vi "I-stat example1.vi"() -> ()   [LabVIEW 2020]
uses:
  SEC Software V3.0/Labview/IVIUM/IVIUM_remdriver.lvlib
panel:
  out "Cell on":bool
  out "C off pressed":bool
  out "E OL":bool
  out "Aninput OL":bool
  out "O overload":bool
  out "Current":dbl
  out "return type":i32
  in  "uA":dbl
  out "potential":dbl
  in  "Stop":bool
  in  "Default\nCurrent range":T1(ring)=enum."100 uA"
  in  "Default Filter":T2(ring)=enum."10 kHz"
  in  "Set Stability":T3(ring)=enum."Standard"
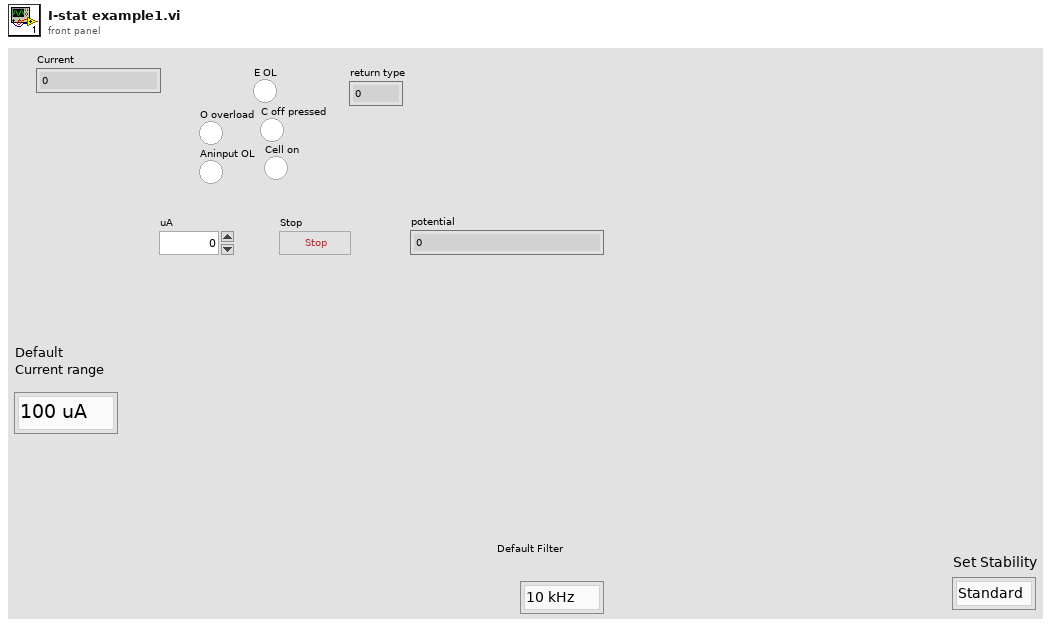
[diagram p1: front panel]
types:
  T1 = enum16{"10 A", "1 A", "100 mA", "10 mA", "1 mA", "100 uA", "10 uA", "1 uA", "100 nA", "10 nA", "1 nA", "100 pA", "10 pA", "1 pA"}
  T2 = enum16{"1 MHz", "100 kHz", "10 kHz", "1 kHz", "10 Hz"}
  T3 = enum16{"High Speed", "Standard", "High Stability"}
  T4 = enum16{"off", "EStat4EL", "EStat2EL", "EStatDummy1", "EStatDummy2", "EStatDummy3", "EStatDummy4", "IStat4EL", "IStat2EL", "IStatDummy", "BiStat4EL", "BiStat2EL"}
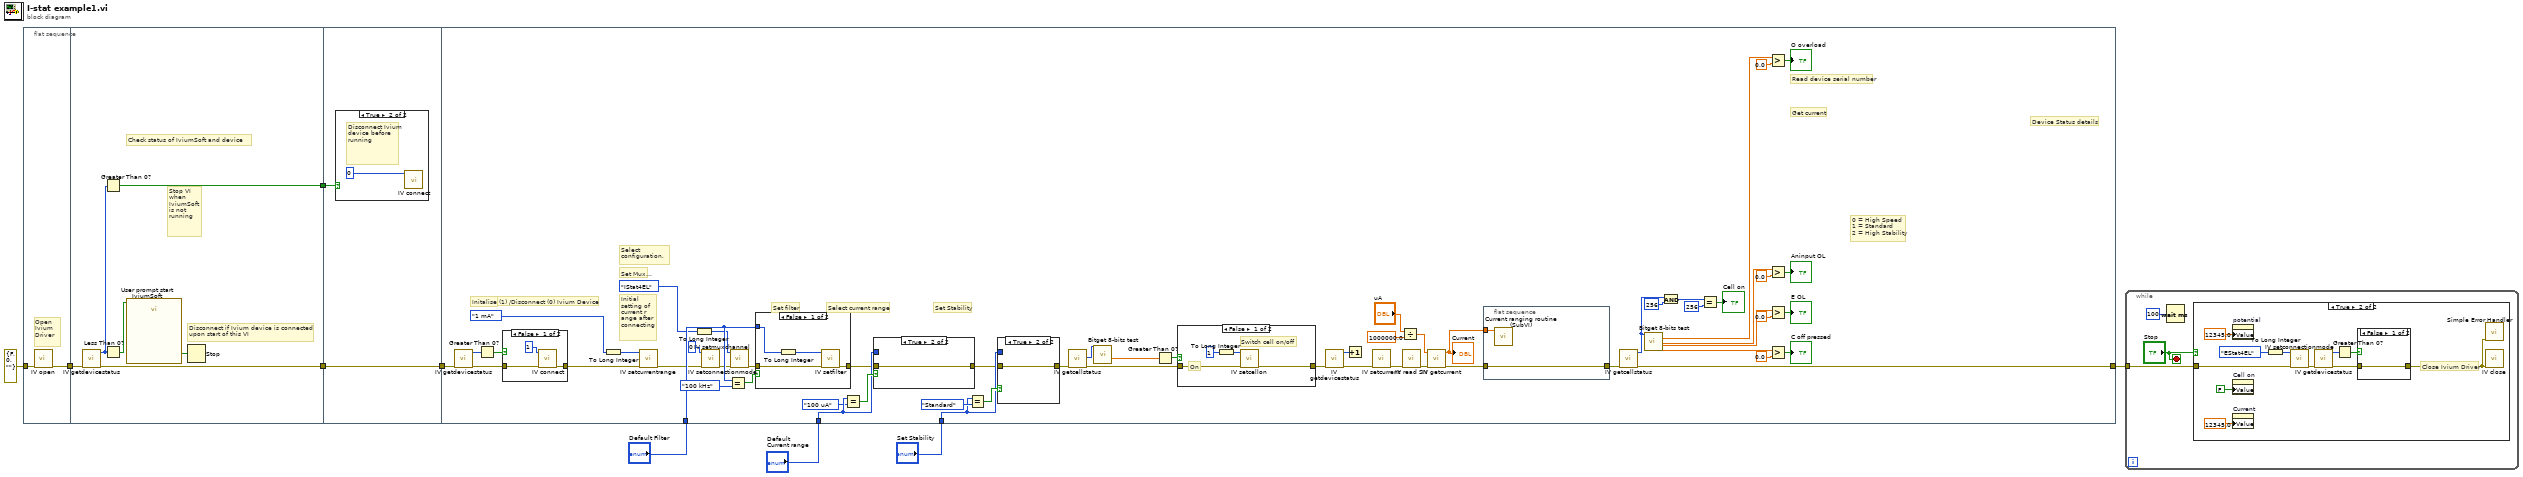
[diagram p0: block diagram]
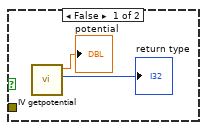
[diagram p2: hidden frame]
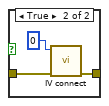
[diagram p3: hidden frame]
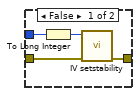
[diagram p7: hidden frame]
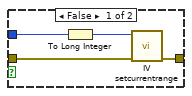
[diagram p9: hidden frame]
diagram:
  n1 = flat-sequence {
    tunnel: [w11] -> w5
    tunnel: errorcluster {"status"=FALSE, "code"=0, "source"=""} ("error in (no error)") -> [w10]
    tunnel: w5 -> [w14]
    tunnel: [w13] -> w4
    tunnel: [w12] -> w3
    tunnel: w4 -> [w19]
    tunnel: [w19] -> w2
    tunnel: w3 -> [w18]
    tunnel: w2 -> [w32]
    tunnel: "Default\nCurrent range" -> [w75]
    tunnel: "Default Filter" -> [w73]
    tunnel: "Set Stability" -> [w71]
    tunnel: [w30] -> w1
    frame #0 {
      # "Open Ivium Driver"
      n2 = call "IV open.vi"("error in (no error)"=w10) -> ("error out"=w11:errorcluster)  [unwired: 9 in, 1 out]
    }
    frame #1 {
      # "Check status of IviumSoft and device"
      # "Stop VI when IviumSoft is not running"
      # "Disconnect if Ivium device is connected \nupon start of this VI"
      n3 = call "IV getdevicestatus.vi"("error in (no error)"=w14) -> ("error out"=w13:errorcluster, "return type"=w17:i32)  [unwired: 9 in]
      n4 = Greater Than 0?(x=w17) -> (x > 0?=w12:bool)
      n5 = Less Than 0?(x=w17) -> (x < 0?=w15:bool)
      n6 = call "User prompt start IviumSoft.vi"("Enable"=w15) -> ("OK"=w16:bool)  [unwired: 17 in, 1 out]
      n7 = Stop(stop? (T)=w16) -> ()
    }
    frame #2 {
      n8 = case shown="True" w18 {
        frame False {
        }
        frame True {
          # "Disconnect Ivium device before running"
          n9 = call "IV connect.vi"("devconnect"=0) -> ()  [unwired: 8 in, 3 out]
        }
      }
    }
    frame #3 {
      # "Device Status details"
      # "Get current"
      # "Set Mux channel"
      # "0 = High Speed\n1 = Standard \n2 = High Stability"
      # "Set Stability"
      # "Set filter"
      # "Select current range"
      # "Select configuration,"
      # "Read device serial number"
      # "Initial setting of current r\nange after connecting"
      # "Connect (1) /Disconnect (0) Ivium Device"
      # "Initalise"
      n10 = call "IV getdevicestatus.vi"("error in (no error)"=w32) -> ("error out"=w44:errorcluster, "return type"=w46:i32)  [unwired: 9 in]
      n11 = Greater Than 0?(x=w46) -> (x > 0?=w45:bool)
      n12 = case shown="False" w45 {
        tunnel: [w83 w84] -> w43
        tunnel: w44 -> [w81 w84]
        frame False {
          n13 = call "IV connect.vi"("error in (no error)"=w81, "devconnect"=1) -> ("error out"=w83:errorcluster)  [unwired: 7 in, 2 out]
        }
        frame True {
        }
      }
      n14 = To Long Integer(number=T1."1 mA" ("Current range selector")) -> (32bit integer=w42:i32)
      n15 = call "IV setcurrentrange.vi"("error in (no error)"=w43, "value"=w42) -> ("error out"=w41:errorcluster)  [unwired: 7 in, 2 out]
      n16 = To Long Integer(number=T4."IStat4EL" ("Configuration")) -> (32bit integer=w39:i32)
      n17 = call "IV setmuxchannel.vi"("error in (no error)"=w41, "value"=0) -> ("error out"=w40:errorcluster)  [unwired: 7 in, 2 out]
      n18 = Equal?(x=w73, y=T2."100 kHz" ("Set Filter")) -> (x = y?=w72:bool)
      n19 = call "IV setconnectionmode.vi"("error in (no error)"=w40, "value"=w39) -> ("error out"=w37:errorcluster)  [unwired: 7 in, 2 out]
      n20 = case shown="False" w72 {
        tunnel: w73 -> [w98 _]
        tunnel: [w96 w99] -> w38
        tunnel: w37 -> [w95 w99]
        frame False {
          n21 = To Long Integer(number=w98) -> (32bit integer=w97:i32)
          n22 = call "IV setfilter.vi"("error in (no error)"=w95, "value"=w97) -> ("error out"=w96:errorcluster)  [unwired: 7 in, 2 out]
        }
        frame True {
        }
      }
      n23 = Equal?(x=w75, y=T1."100 uA") -> (x = y?=w76:bool)
      n24 = case shown="True" w76 {
        tunnel: w75 -> [w102 _]
        tunnel: [w101 w104] -> w36
        tunnel: w38 -> [w100 w104]
        frame False {
          n25 = To Long Integer(number=w102) -> (32bit integer=w103:i32)
          n26 = call "IV setcurrentrange.vi"("error in (no error)"=w100, "value"=w103) -> ("error out"=w101:errorcluster)  [unwired: 7 in, 2 out]
        }
        frame True {
        }
      }
      n27 = Equal?(x=w71, y=T3."Standard" ("Set Stability")) -> (x = y?=w74:bool)
      n28 = case shown="True" w74 {
        tunnel: w71 -> [w93 _]
        tunnel: [w91 w94] -> w35
        tunnel: w36 -> [w90 w94]
        frame False {
          n29 = To Long Integer(number=w93) -> (32bit integer=w92:i32)
          n30 = call "IV setstability.vi"("error in (no error)"=w90, "value"=w92) -> ("error out"=w91:errorcluster)  [unwired: 7 in, 2 out]
        }
        frame True {
        }
      }
      n31 = call "IV getcellstatus.vi"("error in (no error)"=w35) -> ("error out"=w48:errorcluster, "return type"=w52:i32)  [unwired: 8 in, 1 out]
      n32 = call "Bitget 8-bits test.vi"("x"=w52) -> ("f"=w51:dbl)  [unwired: 19 in, 7 out]
      n33 = Greater Than 0?(x=w51) -> (x > 0?=w50:bool)
      n34 = case shown="False" w50 {
        tunnel: w48 -> [w86 w89]
        tunnel: [w85 w89] -> w34
        frame False {
          # "On"
          # "Switch cell on/off"
          n35 = To Long Integer(number=1) -> (32bit integer=w88:i32)
          n36 = call "IV setcellon.vi"("error in (no error)"=w86, "cellon"=w88) -> ("error out"=w85:errorcluster)  [unwired: 7 in, 2 out]
        }
        frame True {
          # "If the cell is already\n on do nothing here"
        }
      }
      n37 = call "IV getdevicestatus.vi"("error in (no error)"=w34) -> ("error out"=w29:errorcluster, "return type"=w69:i32)  [unwired: 9 in]
      n38 = Increment(x=w69) -> ()  [unwired: 1 out]
      n39 = call "IV setcurrent.vi"("error in (no error)"=w29) -> ("error out"=w31:errorcluster)  [unwired: 8 in, 2 out]
      n40 = Divide(x="uA", y=1000000.0) -> (x/y=w23:dbl)
      n41 = call "IV read SN.vi"("error in (no error)"=w31) -> ("error out"=w33:errorcluster)  [unwired: 8 in, 2 out]
      n42 = call "IV getcurrent.vi"("error in (no error)"=w33, "value"=w23) -> ("error out"=w28:errorcluster, "value out"=w26:dbl)  [unwired: 7 in, 1 out]
      "Current" <- w26
      n43 = flat-sequence {
        tunnel: w28 -> [w80]
        tunnel: [w80] -> w27
        tunnel: w26 -> [w79]
        frame #0 {
          n44 = call "Current ranging routine (SubVI).vi"("Current"=w79) -> ()  [unwired: 11 in]
        }
      }
      n45 = call "IV getcellstatus.vi"("error in (no error)"=w27) -> ("error out"=w30:errorcluster, "devcellstatus out"=w60:i32)  [unwired: 8 in, 1 out]
      n46 = call "Bitget 8-bits test.vi"("x"=w60) -> ("c"=w64:dbl, "e"=w62:dbl, "f"=w63:dbl, "h"=w61:dbl)  [unwired: 19 in, 4 out]
      n47 = And(x=w60, y=256) -> (x .and. y?=w58:i32)
      n48 = Equal?(x=w58, y=256) -> (x = y?=→"Cell on":bool)
      n49 = Greater?(x=w64, y=0.0) -> (0:→"O overload":bool)
      n50 = Greater?(x=w62, y=0.0) -> (0:→"Aninput OL":bool)
      n51 = Greater?(x=w63, y=0.0) -> (0:→"E OL":bool)
      n52 = Greater?(x=w61, y=0.0) -> (0:→"C off pressed":bool)
    }
  }
  n53 = while {
    tunnel: w1 -> [w106]
    stop <- "Stop" stop-if-true
    n54 = Wait (ms)(milliseconds to wait=u32 100) -> ()  [unwired: 1 out]
    n55 = case shown="True" "Stop" {
      tunnel: w106 -> [_ w117]
      frame False {
        n56 = call "IV getpotential.vi"() -> ("return type"=→"return type":i32, "value out"=→"potential":dbl)  [unwired: 9 in, 1 out]
      }
      frame True {
        # "Close Ivium Driver"
        n57 = property on="potential" class="DigNum (strict)"("Value"=12345.0 ("potential")) -> ()  [unwired: 2 in, 2 out]
        n58 = property on="Cell on" class="Bool (strict)"("Value"=FALSE ("Cell on")) -> ()  [unwired: 2 in, 2 out]
        n59 = property on="Current" class="DigNum (strict)"("Value"=12345.0 ("Current")) -> ()  [unwired: 2 in, 2 out]
        n60 = To Long Integer(number=T4."EStat4EL" ("Configuration")) -> (32bit integer=w118:i32)
        n61 = call "IV setconnectionmode.vi"("error in (no error)"=w117, "value"=w118) -> ("error out"=w113:errorcluster)  [unwired: 7 in, 2 out]
        n62 = call "IV getdevicestatus.vi"("error in (no error)"=w113) -> ("error out"=w112:errorcluster, "return type"=w114:i32)  [unwired: 9 in]
        n63 = Greater Than 0?(x=w114) -> (x > 0?=w110:bool)
        n64 = case shown="False" w110 {
          tunnel: w112 -> [w121 w123]
          tunnel: [w121 w122] -> w111
          frame False {
          }
          frame True {
            n65 = call "IV connect.vi"("error in (no error)"=w123, "devconnect"=0) -> ("error out"=w122:errorcluster)  [unwired: 7 in, 2 out]
          }
        }
        n66 = call <vilib>:"Simple Error Handler.vi"("error in (no error)"=w111) -> ()  [unwired: 4 in, 5 out]
        n67 = call "IV close.vi"("error in (no error)"=w111) -> ()  [unwired: 9 in, 2 out]
      }
    }
  }
